vi "SetPosition.vi"(8 "error in (no error)":errorcluster caption="entrée d'erreur (pas d'erreur)", 9 "Stop Ref":refnum<vi>, 10 "ScanParIn":dbl, 11 "OR77200 en entrée":refnum<class "OR77200.lvclass"> caption="DNL_LabVIEW Object in") -> (0 "error out":errorcluster caption="sortie d'erreur", 2 "ScanParOut":dbl, 3 "OR77200 en sortie":refnum<class "OR77200.lvclass"> caption="DNL_LabVIEW Object out")   [LabVIEW 2012, in "OR77200.lvclass"]
uses:
  OR77200.lvclass
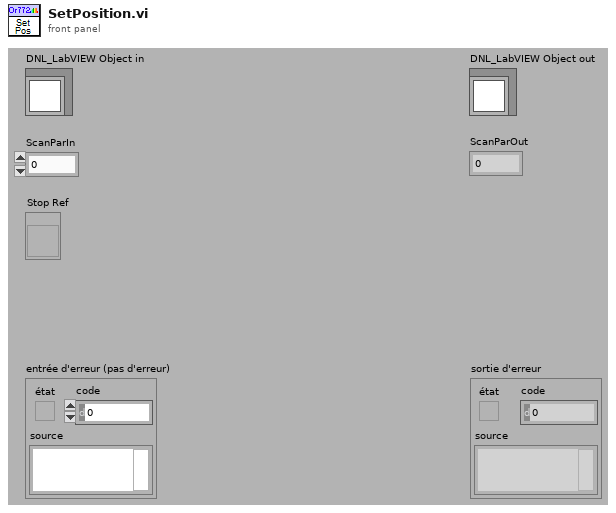
[diagram p1: front panel]
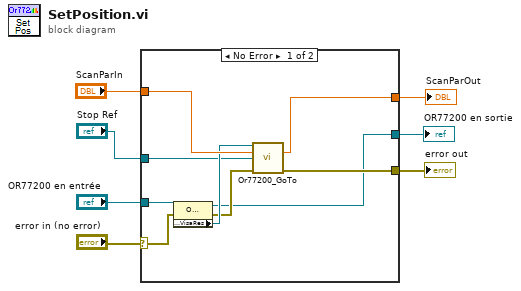
[diagram p0: block diagram]
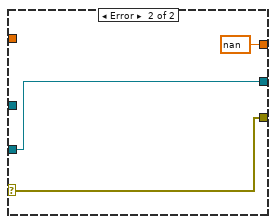
[diagram p2: hidden frame]
diagram:
  n1 = case shown="No Error" "error in (no error)" {
    selector: "error in (no error)" -> [w14 w18]
    tunnel: "ScanParIn" -> [w16 _]
    tunnel: "OR77200 en entrée" -> [w15 w17]
    tunnel: [w11 nan ("Lambda Out (nm)")] -> w4
    tunnel: [w10 w18] -> w3
    tunnel: [w9 w17] -> w2
    tunnel: "Stop Ref" -> [w8 _]
    frame No Error {
      n2 = property class="OR77200.lvclass"(reference=w15, error in=w14) -> (reference out=w9:refnum<class "OR77200.lvclass">, error out=w12:errorcluster, "Accessor:VisaRes"=w13:refnum<visa-resource-name>)
      n3 = call <userlib>:"Or77200_GoTo.vi"("Port"=w13, "Lambda (nm)"=w16, "Stop Ref"=w8, "error In"=w12) -> ("Lambda Out (nm)"=w11:dbl, "sortie d'erreur"=w10:errorcluster)  [unwired: 8 in, 2 out]
    }
    frame Error {
    }
  }
  "error out" <- w3
  "OR77200 en sortie" <- w2
  "ScanParOut" <- w4
